vi "HeapAlloc.vi"(4 "error in (no error)":errorcluster, 5 "Heap Alloc Flags":T1, 6 "dwBytes (1024)":u32=1024, 7 "hHeap (NULL)":i32) -> (0 "error out":errorcluster, 2 "lpMem":i32 format="%.0x", 3 "dup hHeap":i32)   [LabVIEW 2011]
uses:
  KERNEL32.DLL
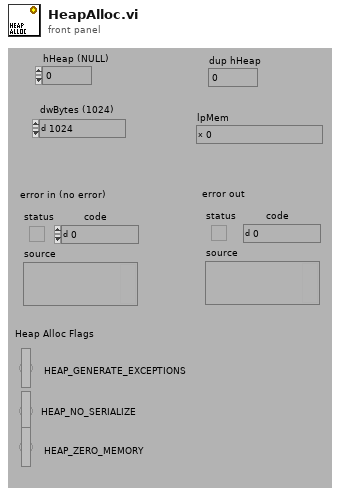
[diagram p1: front panel]
types:
  T1 = cluster{"HEAP_NO_SERIALIZE":bool, "HEAP_GENERATE_EXCEPTIONS":bool, "HEAP_ZERO_MEMORY":bool}
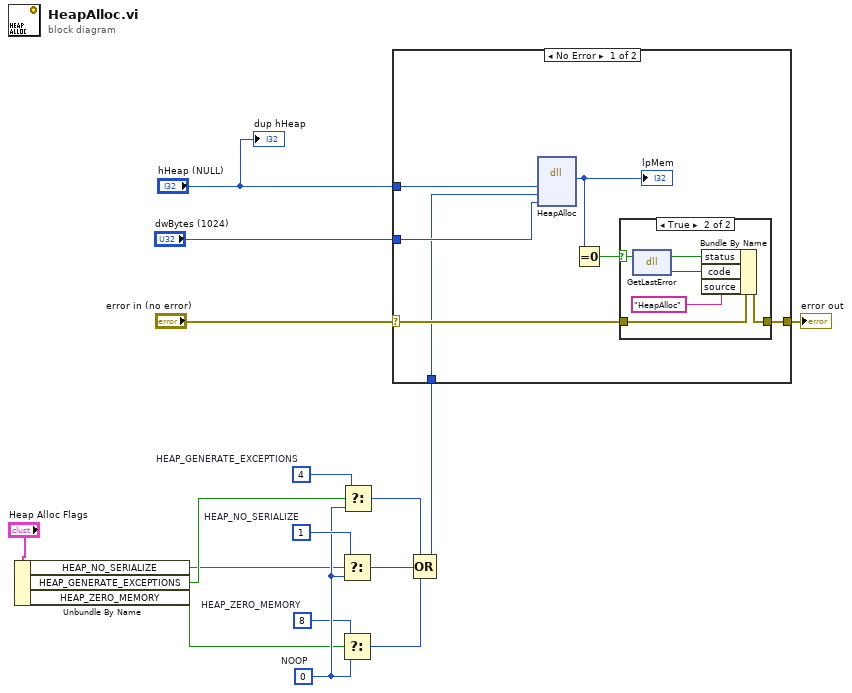
[diagram p0: block diagram]
diagram:
  w6 = u32 8  # HEAP_ZERO_MEMORY
  w8 = u32 0  # NOOP
  w11 = u32 1  # HEAP_NO_SERIALIZE
  w13 = u32 4  # HEAP_GENERATE_EXCEPTIONS
  n1 = Unbundle By Name("Heap Alloc Flags") -> ("HEAP_NO_SERIALIZE"=w3:bool, "HEAP_GENERATE_EXCEPTIONS"=w4:bool, "HEAP_ZERO_MEMORY"=w2:bool)
  n2 = Select(t=w11, s=w3, f=w8) -> (s? t:f=w10:u32)
  n3 = Select(t=w6, s=w2, f=w8) -> (s? t:f=w9:u32)
  n4 = Select(t=w13, s=w4, f=w8) -> (s? t:f=w12:u32)
  n5 = Compound Arithmetic op=OR(w12, w10, w9) -> (w7:u32)
  n6 = case shown="No Error" "error in (no error)" {
    selector: "error in (no error)" -> [w21 w30]
    tunnel: [w20 w30] -> w15
    tunnel: "dwBytes (1024)" -> [w19 _]
    tunnel: w7 -> [w18 _]
    tunnel: "hHeap (NULL)" -> [w17 _]
    frame No Error {
      n7 = dll-call lib="KERNEL32.DLL" fn="HeapAlloc" label="LPVOID HeapAlloc(\n  HANDLE hHeap,   // handle to private heap block\n  DWORD dwFlags,  // heap allocation control\n  SIZE_T dwBytes  // number of bytes to allocate\n);"("hHeap"=w17, "dwFlags"=w18, "dwBytes"=w19) -> ("lpMem"=w23:i32)  [unwired: 6 in, 2 out]
      "lpMem" <- w23
      n8 = Equal To 0?(x=w23) -> (x = 0?=w22:bool)
      n9 = case shown="True" w22 {
        selector: w22 -> [_ w28]
        tunnel: w21 -> [w24 w29]
        tunnel: [w24 w27] -> w20
        frame False {
        }
        frame True {
          n10 = dll-call lib="KERNEL32.DLL" fn="GetLastError"() -> (w26:i32)  [unwired: 3 in, 2 out]
          n11 = Bundle By Name(cluster=w29, "status"=w28, "code"=w26, "source"="HeapAlloc") -> (w27:errorcluster)
        }
      }
    }
    frame Error {
    }
  }
  "error out" <- w15
  "dup hHeap" <- "hHeap (NULL)"
